vi "Quick Sort 2D Coordinates.vi"(4 "2D Coordinates":cluster{"x1":dbl, "x2":dbl}[](array[cluster])) -> (1 "Sorted 2D Coordinates":cluster{"x1":dbl, "x2":dbl}[](array[cluster]))   [LabVIEW 2013]
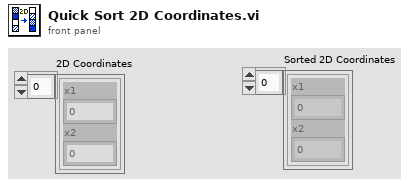
[diagram p1: front panel]
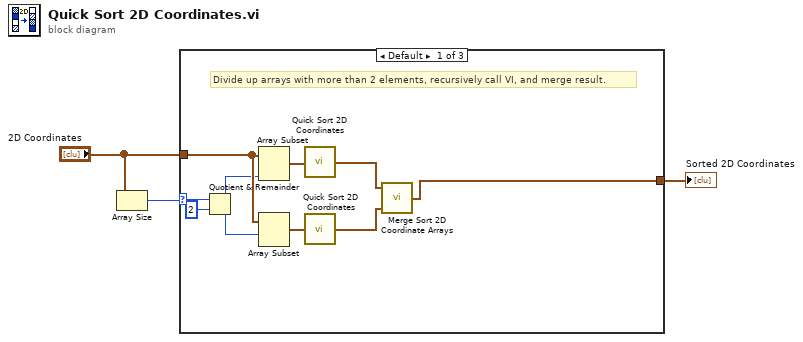
[diagram p0: block diagram]
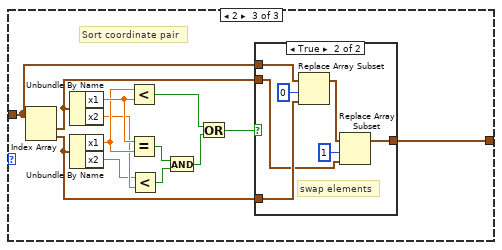
[diagram p3: hidden frame]
diagram:
  n1 = Array Size(array="2D Coordinates") -> (size(s)=w3:i32)
  n2 = case shown="Default" w3 {
    selector: w3 -> [w12 _ _]
    tunnel: "2D Coordinates" -> [w10 w13 w17]
    tunnel: [w4 w13 w15] -> w1
    frame Default {
      # "Divide up arrays with more than 2 elements, recursively call VI, and merge result."
      n3 = Quotient & Remainder(x=w12, y=2) -> (floor(x/y)=w9:i32)  [unwired: 1 out]
      n4 = Array Subset(array=w10, length=w9) -> (w8:cluster{"x1":dbl, "x2":dbl}[])  [unwired: 1 in]
      n5 = Array Subset(array=w10, index=w9) -> (w7:cluster{"x1":dbl, "x2":dbl}[])  [unwired: 1 in]
      n6 = call "Quick Sort 2D Coordinates.vi"("2D Coordinates"=w8) -> ("Sorted 2D Coordinates"=w6:cluster{"x1":dbl, "x2":dbl}[])  [unwired: 4 in]
      n7 = call "Quick Sort 2D Coordinates.vi"("2D Coordinates"=w7) -> ("Sorted 2D Coordinates"=w5:cluster{"x1":dbl, "x2":dbl}[])  [unwired: 4 in]
      n8 = call "Merge Sort 2D Coordinate Arrays.vi"("2D Coordinate Array A"=w6, "2D Coordinate Array B"=w5) -> ("Sorted 2D Coordinate Array"=w4:cluster{"x1":dbl, "x2":dbl}[])  [unwired: 5 in]
    }
    frame 0, 1 {
      # "Pass through single elements."
    }
    frame 2 {
      # "Sort coordinate pair"
      n9 = Index Array(array=w17) -> (element #1=w16:cluster{"x1":dbl, "x2":dbl}, element #2=w18:cluster{"x1":dbl, "x2":dbl})  [unwired: 2 in]
      n10 = Unbundle By Name(w16) -> ("x1"=w25:dbl, "x2"=w21:dbl)
      n11 = Unbundle By Name(w18) -> ("x1"=w24:dbl, "x2"=w20:dbl)
      n12 = Less?(x=w24, y=w25) -> (x < y?=w26:bool)
      n13 = Equal?(x=w25, y=w24) -> (x = y?=w23:bool)
      n14 = Less?(x=w20, y=w21) -> (x < y?=w22:bool)
      n15 = And(x=w23, y=w22) -> (x .and. y?=w19:bool)
      n16 = Or(x=w26, y=w19) -> (x .or. y?=w14:bool)
      n17 = case shown="True" w14 {
        tunnel: w18 -> [_ w33]
        tunnel: w17 -> [w27 w32]
        tunnel: w16 -> [_ w30]
        tunnel: [w27 w28] -> w15
        frame False {
        }
        frame True {
          # "swap elements"
          n18 = Replace Array Subset(array=w32, new element=w33, index=0) -> (w29:cluster{"x1":dbl, "x2":dbl}[])
          n19 = Replace Array Subset(array=w29, new element=w30, index=1) -> (w28:cluster{"x1":dbl, "x2":dbl}[])
        }
      }
    }
  }
  "Sorted 2D Coordinates" <- w1
